vi "AFG Report Event.vi"(8 "error in (no error)":errorcluster, 9 "Event Data":variant, 10 "Report Events":T1=enum."Inited", 11 "Controller in":refnum<class "Controller.lvclass">) -> (0 "error out":errorcluster, 3 "Controller out":refnum<class "Controller.lvclass">)   [LabVIEW 2020, in "Controller.lvlib" / "Controller.lvclass"]
uses:
  Controller.lvclass
  C:/Program Files/National Instruments/LabVIEW 2020/vi.lib/ActorFramework/Actor/Actor.lvclass
  Actor_AFG/AFG_Event.ctl
  <vilib>/ActorFramework/Actor/Actor.lvclass/Actor.ctl
  <vilib>/ActorFramework/Message Enqueuer/Message Enqueuer.lvclass/Message Enqueuer.ctl
  Controller.lvclass/Controller.ctl
  Actor_log/Actor_log Messages/Write Event to Log Msg/Write Event to Log Msg.lvclass/Write Event to Log Msg.ctl
  <vilib>/ActorFramework/Message Enqueuer/Init from Existing Queue.vi
  <vilib>/ActorFramework/Message Enqueuer/Enqueue.vi
  <vilib>/ActorFramework/Stop Msg/Send Emergency Stop.vi
  <vilib>/ActorFramework/Stop Msg/Send Normal Stop.vi
  <vilib>/ActorFramework/Message Enqueuer/Enqueue Critical.vi
  Actor_log/Actor_log Messages/Write Event to Log Msg/Write Event to Log Msg.lvclass
  C:/Program Files/National Instruments/LabVIEW 2020/vi.lib/ActorFramework/Message/Message.lvclass
  <vilib>/ActorFramework/Stop Msg/Stop Msg.lvclass
  <vilib>/ActorFramework/Message Priority Queue/Priority Enqueue.vi
  <vilib>/ActorFramework/Message Enqueuer/Message Enqueuer.lvclass
  <vilib>/ActorFramework/Actor/Actor.lvclass
  Actor_AFG/Actor_AFG/Actor_AFG.lvclass
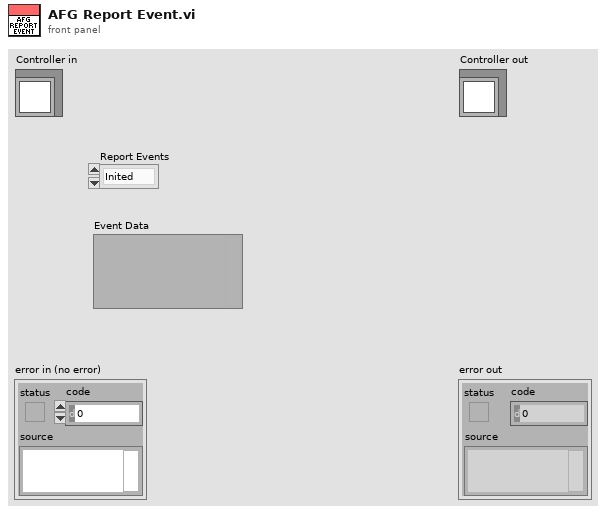
[diagram p1: front panel]
types:
  T1 = typedef "Actor_AFG.lvlib/Actor_AFG.lvclass/AFG_Event.ctl" = enum16{"General Event", "Inited", "Output", "Waveform Set", "DC Configured", "Cycle End", "Error"}
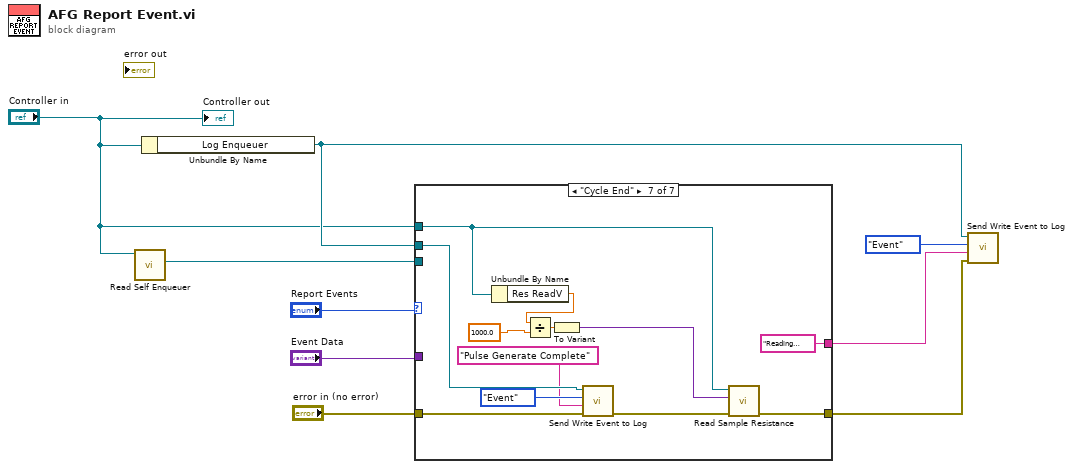
[diagram p0: block diagram]
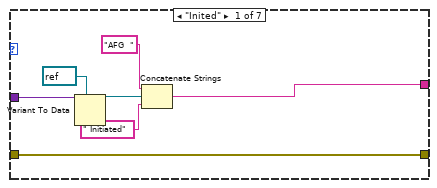
[diagram p2: hidden frame]
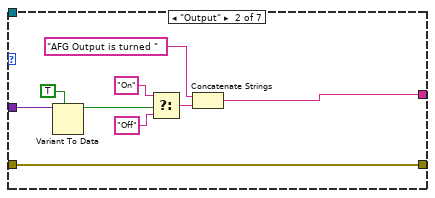
[diagram p3: hidden frame]
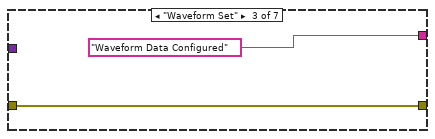
[diagram p4: hidden frame]
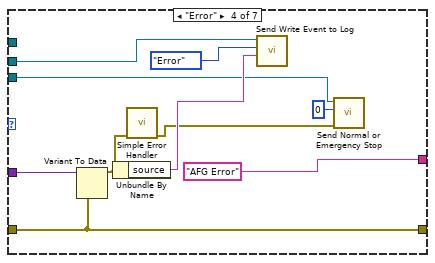
[diagram p5: hidden frame]
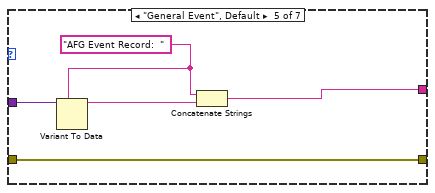
[diagram p6: hidden frame]
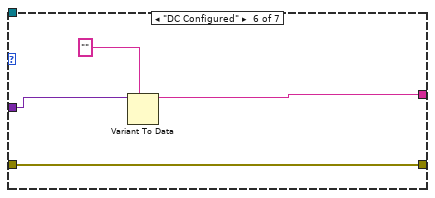
[diagram p7: hidden frame]
diagram:
  n1 = call <vilib>:"Read Self Enqueuer.vi"("Actor"="Controller in") -> ("Self Enqueuer"=w6:refnum<class "Message Enqueuer.lvclass">)  [unwired: 10 in]
  n2 = Unbundle By Name("Controller in") -> ("Log Enqueuer"=w4:refnum<class "Message Enqueuer.lvclass">)
  n3 = case shown="\"Cycle End\"" "Report Events" {
    tunnel: "Event Data" -> [w16 w24 _ w36 w40 w44 _]
    tunnel: "error in (no error)" -> [w11 w25 w27 w37 w42 w46 w57]
    tunnel: [w11 w25 w27 w37 w42 w46 w54] -> w2
    tunnel: [w10 w17 "Waveform Data Configured" "AFG Error" w38 w43 "Reading Sample Resistance"] -> w3
    tunnel: w4 -> [_ _ _ w31 _ _ w56]
    tunnel: w6 -> [_ _ _ w29 _ _ _]
    tunnel: "Controller in" -> [_ _ _ _ _ _ w52]
    frame "Inited" {
      n4 = Variant To Data(type=refnum<visa-resource-name> refnum ("VISA resource name"), Variant=w16) -> (data=w14:refnum<visa-resource-name>)  [unwired: 1 in, 1 out]
      n5 = Concatenate Strings("AFG  " ("string"), w14, " Initiated" ("string")) -> (w10:string)
    }
    frame "Output" {
      n6 = Variant To Data(type=TRUE, Variant=w24) -> (data=w22:bool)  [unwired: 1 in, 1 out]
      n7 = Select(t="On", s=w22, f="Off") -> (s? t:f=w19:string)
      n8 = Concatenate Strings("AFG Output is turned ", w19) -> (w17:string)
    }
    frame "Waveform Set" {
    }
    frame "Error" {
      n9 = Variant To Data(type=w37, Variant=w36) -> (data=w33:errorcluster)  [unwired: 1 in, 1 out]
      n10 = Unbundle By Name(w33) -> ("source"=w32:string)
      n11 = call <vilib>:"Simple Error Handler.vi"("error in (no error)"=w33) -> ("error out"=w28:errorcluster)  [unwired: 4 in, 4 out]
      n12 = call "Send Write Event to Log.vi"("Log Event Details"=w32, "Enum"=enum16{"Event", "Error"}."Error", "Message Enqueuer"=w31) -> ()  [unwired: 7 in, 2 out]
      n13 = call <vilib>:"Send Normal or Emergency Stop.vi"("error in (no error)"=w28, "final error code"=0, "Message Enqueuer"=w29) -> ()  [unwired: 8 in, 1 out]
    }
    frame "General Event", Default {
      w41 = "AFG Event Record:  "
      n14 = Variant To Data(type=w41, Variant=w40) -> (data=w39:string)  [unwired: 1 in, 1 out]
      n15 = Concatenate Strings(w41, w39) -> (w38:string)
    }
    frame "DC Configured" {
      n16 = Variant To Data(type="", Variant=w44) -> (data=w43:string)  [unwired: 1 in, 1 out]
    }
    frame "Cycle End" {
      n17 = Unbundle By Name(w52) -> ("Res ReadV"=w48:dbl)
      n18 = Divide(x=w48, y=1000.0) -> (x/y=w49:dbl)
      n19 = To Variant(anything=w49) -> (Variant=w53:variant)
      n20 = call "Send Write Event to Log.vi"("error in (no error)"=w57, "Log Event Details"="Pulse Generate Complete", "Enum"=enum16{"Event", "Error"}."Event", "Message Enqueuer"=w56) -> ("error out"=w55:errorcluster)  [unwired: 6 in, 1 out]
      n21 = call-dynamic "Read Sample Resistance.vi"("error in (no error)"=w55, "Action Data"=w53, "Controller in"=w52) -> ("error out"=w54:errorcluster)  [unwired: 7 in, 1 out]
    }
  }
  n22 = call "Send Write Event to Log.vi"("error in (no error)"=w2, "Log Event Details"=w3, "Enum"=enum16{"Event", "Error"}."Event", "Message Enqueuer"=w4) -> ()  [unwired: 6 in, 2 out]
  "Controller out" <- "Controller in"
